vi "Count Event Message by Message.vi"(8 "error in (no error)":errorcluster, 9 "Timeout":i32, 10 "Message":T1, 11 "Event Registration Refnum in":refnum<event-registration>) -> (0 "error out":errorcluster, 1 "Message Data":variant[](array[variant]), 2 "Count":i32, 3 "Event Registration Refnum out":refnum<event-registration>)   [LabVIEW 2020, in "Process Test.lvclass"]
uses:
  Process Test.lvclass
  Framework/Process/Protected/Broadcasting/Broadcast Message Cluster.ctl
  Framework/Broadcast Event Helpers/Execution timer.vi
  Framework/Broadcast Event Helpers/Dequeue Broadcast Message.vi
  Process Test.lvclass/Process Test.ctl
  Framework/Broadcast Event Helpers/Broadcast Event Helpers.lvlib
  Framework/Process/Process.lvclass
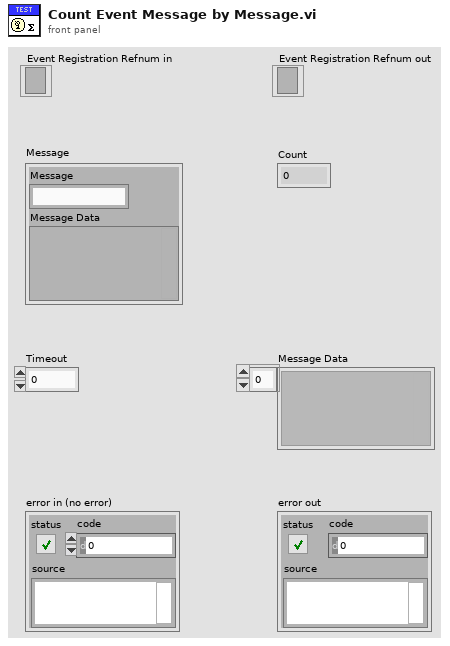
[diagram p1: front panel]
types:
  T1 = cluster{"Message":string, "Message Data":variant}
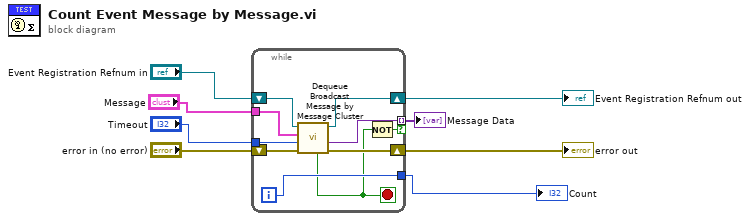
[diagram p0: block diagram]
diagram:
  n1 = while {
    tunnel: "Timeout" -> [w17]
    shift-right: [w18] -> w8
    shift-left: "error in (no error)" -> [w16]
    shift-right: [w15] -> w5
    shift-left: "Event Registration Refnum in" -> [w14]
    tunnel: [w13] -> w3
    tunnel: [w12] -> w2 mode=indexing if=w10
    tunnel: "Message" -> [w9]
    i -> [w13]
    stop <- w11 stop-if-true
    n2 = call "Dequeue Broadcast Message by Message Cluster.vi"("error in (no error)"=w16, "Timeout (-1)"=w17, "Message"=w9, "Event Registration Refnum"=w14) -> ("error out"=w18:errorcluster, "Message Data"=w12:variant, "Event Registration Refnum Out"=w15:refnum<event-registration>, "Timed Out?"=w11:bool)  [unwired: 3 in, 1 out]
    n3 = Not(x=w11) -> (.not. x?=w10:bool)
  }
  "error out" <- w8
  "Event Registration Refnum out" <- w5
  "Count" <- w3
  "Message Data" <- w2
